vi "Curtin1_suggestTestName.vi"(10 "instrument":string, 11 "Build?":bool=TRUE) -> (2 "Suggested Test":string)   [LabVIEW 2022 SP3]
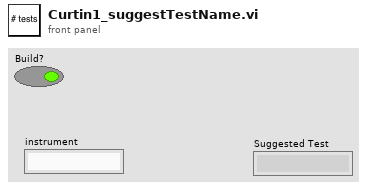
[diagram p1: front panel]
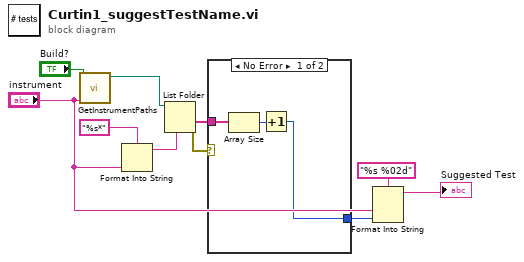
[diagram p0: block diagram]
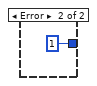
[diagram p2: hidden frame]
diagram:
  n1 = call "GetInstrumentPaths.vi"("Instrument"="instrument", "Build?"="Build?") -> ("Path To Instrument Folder"=w7:path)  [unwired: 5 in, 4 out]
  n2 = Format Into String(format string="%s*" ("name or relative path"), "instrument") -> (resulting string=w9:string)  [unwired: 2 in, 1 out]
  n3 = List Folder(path=w7, pattern=w9) -> (folder names=w10:string[], error out=w2:errorcluster)  [unwired: 2 in, 2 out]
  n4 = case shown="No Error" w2 {
    tunnel: w10 -> [w13 _]
    tunnel: [w11 1] -> w3
    frame No Error {
      n5 = Array Size(array=w13) -> (size(s)=w12:i32)
      n6 = Increment(x=w12) -> (x+1=w11:i32)
    }
    frame Error {
    }
  }
  n7 = Format Into String(format string="%s %02d", "instrument", w3) -> (resulting string=→"Suggested Test":string)  [unwired: 2 in, 1 out]
